vi "Periodic gate function.vi"(1 "# of samples":dbl=100.0, 2 "Time period (T)":dbl=10.0, 3 "width":dbl=5.0, 4 "Amplitude":dbl=1.0) -> (0 "Pulse gate":dbl[](array[numeric])=[1.0, 1.0, 1.0, 1.0, 1.0, 0.0, 0.0, 0.0, 0.0, 0.0, 0.0, 0.0, 0.0, 0.0, 0.0, 0.0, 0.0, 0.0, 0.0, 0.0, 1.0, 1.0, 1.0, 1.0, 1.0, 0.0, 0.0, 0.0, 0.0, 0.0, 0.0, 0.0, 0.0, 0.0, 0.0, 0.0, 0.0, 0.0, 0.0, 0.0, 1.0, 1.0, 1.0, 1.0, 1.0, 0.0, 0.0, 0.0, 0.0, 0.0, 0.0, 0.0, 0.0, 0.0, 0.0, 0.0, 0.0, 0.0, 0.0, 0.0, 1.0, 1.0, 1.0, 1.0, 1.0, 0.0, 0.0, 0.0, 0.0, 0.0, 0.0, 0.0, 0.0, 0.0, 0.0, 0.0, 0.0, 0.0, 0.0, 0.0, 1.0, 1.0, 1.0, 1.0, 1.0, 0.0, 0.0, 0.0, 0.0, 0.0, 0.0, 0.0, 0.0, 0.0, 0.0, 0.0, 0.0, 0.0, 0.0, 0.0, 1.0, 1.0, 1.0, 1.0, 1.0, 0.0, 0.0, 0.0, 0.0, 0.0, 0.0, 0.0, 0.0, 0.0, 0.0, 0.0, 0.0, 0.0, 0.0, 0.0, 1.0, 1.0, 1.0, 1.0, 1.0, 0.0, 0.0, 0.0, 0.0, 0.0, 0.0, 0.0, 0.0, 0.0])   [LabVIEW 2009]
uses:
  <vilib>/Analysis/NI_AALBase.lvlib
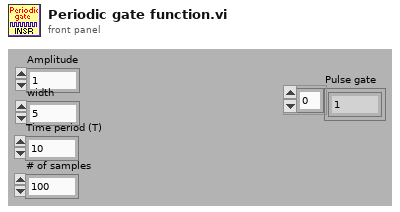
[diagram p1: front panel]
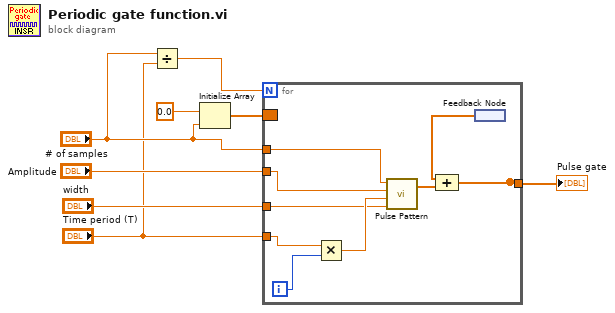
[diagram p0: block diagram]
diagram:
  n1 = Divide(x="# of samples", y="Time period (T)") -> (x/y=w2:dbl)
  n2 = Initialize Array(0.0 ("element"), "# of samples") -> (w5:dbl[])
  n3 = for {
    N: w2 -> [_]
    tunnel: "Time period (T)" -> [w16]
    tunnel: "width" -> [w14]
    tunnel: "Amplitude" -> [w13]
    tunnel: "# of samples" -> [w12]
    tunnel: [w9] -> w1
    border: w5 -> [_]
    i -> [w17]
    n4 = Multiply(x=w16, y=w17) -> (x*y=w15:dbl)
    n5 = call <vilib>:"Pulse Pattern.vi"("width"=w14, "delay"=w15, "amplitude"=w13, "samples"=w12) -> ("Pulse Pattern"=w11:dbl[])  [unwired: 1 out]
    n6 = feedback #1() -> (w10:dbl[])
    n7 = Compound Arithmetic op=ADD(w10, w11) -> (w9:dbl[])
  }
  "Pulse gate" <- w1
